vi "Parallel Derivative Calculation.vi"(6 "alpha":dbl=nan, 8 "dt":dbl, 9 "Reinit":bool, 10 "process variable in":dbl, 11 "PID gains":T1) -> (2 "deriv Term":dbl)   [LabVIEW 2020]
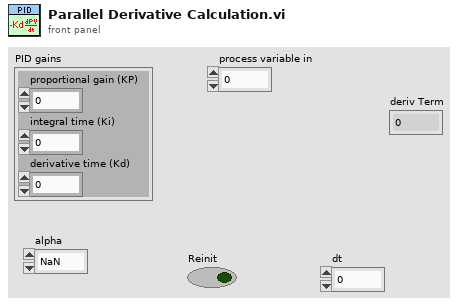
[diagram p1: front panel]
types:
  T1 = cluster{"proportional gain (KP)":dbl, "integral time (Ki)":dbl, "derivative time (Kd)":dbl}
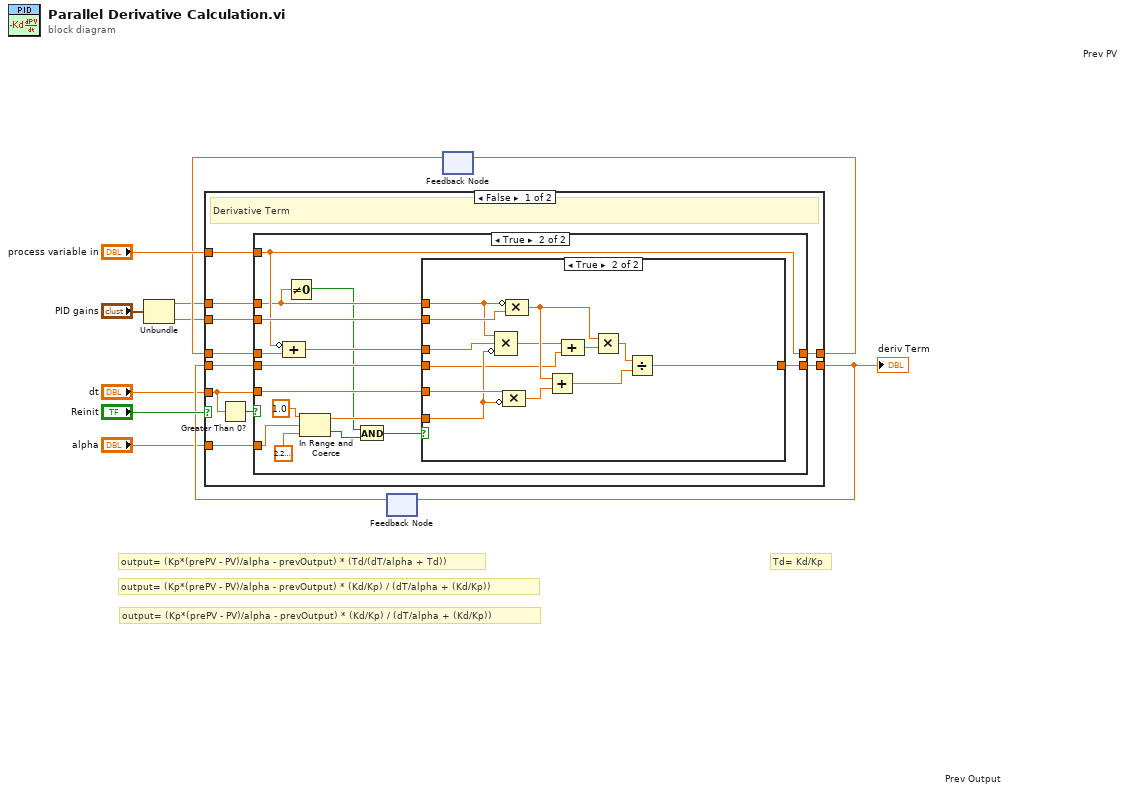
[diagram p0: block diagram]
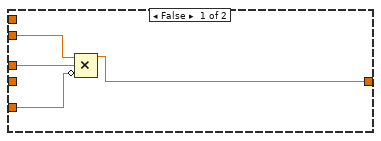
[diagram p3: hidden frame]
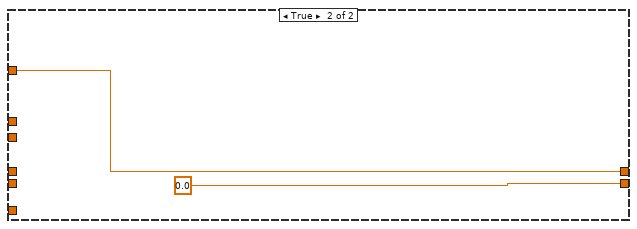
[diagram p4: hidden frame]
diagram:
  # "output= (Kp*(prePV - PV)/alpha - prevOutput) * (Kd/Kp) / (dT/alpha + (Kd/Kp))"
  # "Td= Kd/Kp"
  # "output= (Kp*(prePV - PV)/alpha - prevOutput) * (Kd/Kp) / (dT/alpha + (Kd/Kp))"
  # "output= (Kp*(prePV - PV)/alpha - prevOutput) * (Td/(dT/alpha + Td))"
  n1 = Unbundle("PID gains") -> ("proportional gain (KP)"=w3:dbl, "derivative time (Kd)"=w4:dbl)  [unwired: 1 out]
  n2 = feedback #1 "Prev Output"() -> (w6:dbl)  [unwired: 1 in]
  n3 = feedback #2 "Prev PV"() -> (w5:dbl)  [unwired: 1 in]
  n4 = case shown="False" "Reinit" {
    tunnel: w5 -> [w21 _]
    tunnel: w4 -> [w18 _]
    tunnel: "process variable in" -> [w20 w57]
    tunnel: [w17 w57] -> w9
    tunnel: [w19 0.0] -> w7
    tunnel: w6 -> [w15 _]
    tunnel: "dt" -> [w14 _]
    tunnel: w3 -> [w13 _]
    tunnel: "alpha" -> [w12 _]
    frame False {
      # "Derivative Term"
      n5 = Greater Than 0?(x=w14) -> (x > 0?=w16:bool)
      n6 = case shown="True" w16 {
        tunnel: w21 -> [w23 w34]
        tunnel: w14 -> [_ w37]
        tunnel: w20 -> [_ w35]
        tunnel: [w22 w36] -> w19
        tunnel: w18 -> [_ w38]
        tunnel: [w23 w35] -> w17
        tunnel: w15 -> [w22 w32]
        tunnel: w13 -> [_ w27]
        tunnel: w12 -> [_ w30]
        frame False {
          # "dt = 0 min"
        }
        frame True {
          n7 = Compound Arithmetic op=ADD(invert w35, w34) -> (w33:dbl)
          n8 = Not Equal To 0?(x=w27) -> (x != 0?=w26:bool)
          n9 = In Range and Coerce(upper limit=1.0 ("lower limit"), x=w30, lower limit=2.220446049250313e-16) -> (coerced(x)=w28:dbl, In Range?=w25:bool)
          n10 = And(x=w26, y=w25) -> (x .and. y?=w24:bool)
          n11 = case shown="True" w24 {
            tunnel: w38 -> [w42 w55]
            tunnel: w37 -> [w41 w53]
            tunnel: [w40 w43] -> w36
            tunnel: w28 -> [_ w46]
            tunnel: w33 -> [w39 w47]
            tunnel: w32 -> [_ w44]
            tunnel: w27 -> [_ w45]
            frame False {
              n12 = Compound Arithmetic op=MULTIPLY(w42, w39, invert w41) -> (w40:dbl)
            }
            frame True {
              n13 = Compound Arithmetic op=MULTIPLY(w45, w47, invert w46) -> (w48:dbl)
              n14 = Compound Arithmetic op=MULTIPLY(w53, invert w46) -> (w52:dbl)
              n15 = Compound Arithmetic op=MULTIPLY(invert w45, w55) -> (w51:dbl)
              n16 = Add(x=w51, y=w52) -> (x+y=w49:dbl)
              n17 = Compound Arithmetic op=ADD(w48, w44) -> (w54:dbl)
              n18 = Multiply(x=w51, y=w54) -> (x*y=w50:dbl)
              n19 = Divide(x=w50, y=w49) -> (x/y=w43:dbl)
            }
          }
        }
      }
    }
    frame True {
    }
  }
  "deriv Term" <- w7
  n20 = feedback-in #1(w7) -> ()
  n21 = feedback-in #2(w9) -> ()
